vi "Check File Size.vi"(8 "error in (no error)":errorcluster, 11 "[M] TDMS Save in":refnum<class "[M] TDMS Save.lvclass">) -> (0 "error out":errorcluster, 3 "[M] TDMS Save out":refnum<class "[M] TDMS Save.lvclass">)   [LabVIEW 2023, in "[M] TDMS Save.lvlib" / "[M] TDMS Save.lvclass"]
uses:
  [M] TDMS Save.lvclass
  [M] TDMS Save.lvclass/[M] TDMS Save.ctl
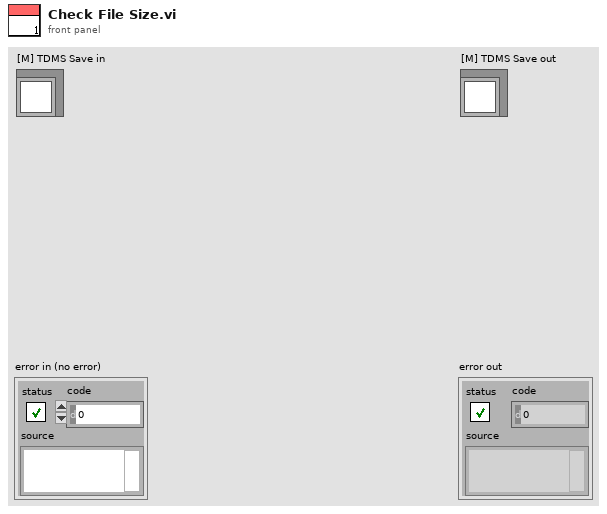
[diagram p1: front panel]
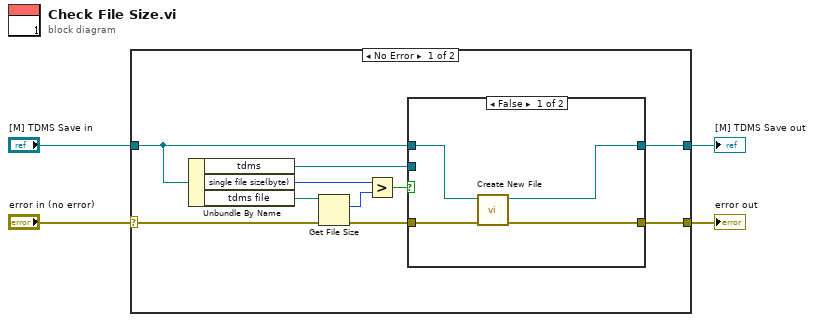
[diagram p0: block diagram]
diagram:
  n1 = case shown="No Error" "error in (no error)" {
    selector: "error in (no error)" -> [w14 w22]
    tunnel: [w5 w22] -> w3
    tunnel: [w6 w21] -> w1
    tunnel: "[M] TDMS Save in" -> [w10 w21]
    frame No Error {
      n2 = Unbundle By Name(w10) -> ("tdms"=w7:refnum<k34>, "single file size(byte)"=w12:i64, "tdms file"=w13:path)
      n3 = Get File Size(file=w13, error in=w14) -> (size (in bytes)=w11:i64, 0:w8:errorcluster)  [unwired: 1 out]
      n4 = Greater?(x=w12, y=w11) -> (0:w9:bool)
      n5 = case shown="False" w9 {
        tunnel: w10 -> [w17 w20]
        tunnel: w8 -> [w18 w19]
        tunnel: w7 -> [_ _]
        tunnel: [w15 w20] -> w6
        tunnel: [w16 w19] -> w5
        frame False {
          n6 = call "Create New File.vi"("error in (no error)"=w18, "[M] TDMS Save in"=w17) -> ("error out"=w16:errorcluster, "[M] TDMS Save out"=w15:refnum<class "[M] TDMS Save.lvclass">)  [unwired: 8 in]
        }
        frame True {
        }
      }
    }
    frame Error {
    }
  }
  "error out" <- w3
  "[M] TDMS Save out" <- w1
